vi "LorentzianMOD.vi"(3 "output control":T1, 4 "data":variant, 5 "X":dbl[](array[numeric]), 6 "a":dbl[](array[numeric])) -> (0 "error out":errorcluster, 1 "f'(X,a)":dbl[][](array[numeric]), 2 "f(x,a)":dbl[](array[numeric]))   [LabVIEW 2017]
uses:
  <vilib>/gmath/NumericalOptimization/LM_output select.ctl
  <vilib>/gmath/NI_Gmath.lvlib
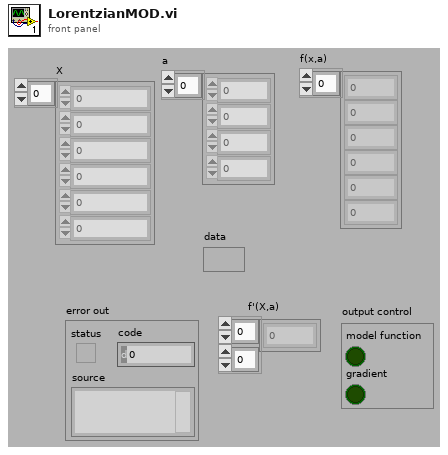
[diagram p1: front panel]
types:
  T1 = typedef "NI_Gmath.lvlib/LM_output select.ctl" = cluster{"model function":bool, "gradient":bool}
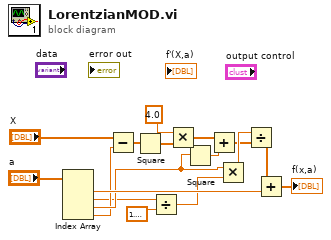
[diagram p0: block diagram]
diagram:
  n1 = Index Array(array="a") -> (element #1=w15:dbl, element #2=w1:dbl, element #3=w14:dbl, element #4=w13:dbl)  [unwired: 4 in]
  n2 = Subtract(x="X", y=w13) -> (x-y=w9:dbl[])
  n3 = Square(x=w9) -> (x^2=w8:dbl[])
  n4 = Divide(x=w1, y=1.5707963267948966) -> (x/y=w10:dbl)
  n5 = Multiply(x=4.0, y=w8) -> (x*y=w6:dbl[])
  n6 = Square(x=w14) -> (x^2=w5:dbl)
  n7 = Add(x=w6, y=w5) -> (x+y=w3:dbl[])
  n8 = Multiply(x=w14, y=w10) -> (x*y=w4:dbl)
  n9 = Divide(x=w4, y=w3) -> (x/y=w2:dbl[])
  n10 = Add(x=w2, y=w15) -> (x+y=→"f(x,a)":dbl[])
